vi "Boolean Trigger.vi"(10 "Value":bool, 11 "Reset":bool) -> (2 "Value out":bool)   [LabVIEW 2018]
uses:
  <instrlib>/_niInstr/Basic Elements/v1/FPGA/niInstr Basic Elements v1 FPGA.lvlib
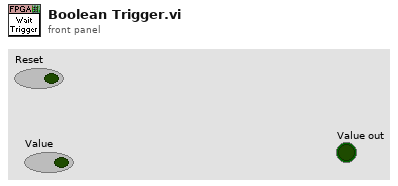
[diagram p1: front panel]
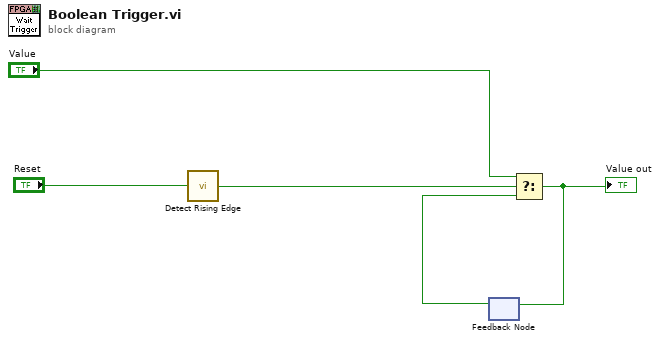
[diagram p0: block diagram]
diagram:
  n1 = call <instrlib>:"Detect Rising Edge.vi"("signal"="Reset") -> ("edge detected"=w3:bool)  [unwired: 14 in]
  n2 = feedback #1() -> (w1:bool)  [unwired: 1 in]
  n3 = Select(t="Value", s=w3, f=w1) -> (s? t:f=w5:bool)
  "Value out" <- w5
  n4 = feedback-in #1(w5) -> ()
